vi "Deserialize Data.vi"(8 "error in (no error)":errorcluster, 11 "Flat Data in":string) -> (0 "error out":errorcluster, 3 "Process Data out":T1 {"CAN Frame Array"."payload" format="%x"; "CAN Frame Array"."timestamp" format="%<%.7X\n%x>T"; "CAN Frame Array"."type" items=["CAN Data"=0, "CAN Remote"=1, "CAN Bus Error"=2, "CAN 2.0 Data"=8, "CAN FD Data"=16, "CAN FD+BRS Data"=24, "J1939 Data"=192, "Delay"=224, "Log Trigger"=225, "Start Trigger"=226]; "CAN Frame Array"."identifier" format="%x"})   [LabVIEW 2020, in "NI_ADAS_CAN.lvlib"]
doc: "Version 0.1"
uses:
  NI_ADAS_CAN.lvlib
  Process Data.ctl
  <vilib>/xnet/xnet.llb/XNET Frame CAN.ctl
  <vilib>/xnet/xnet.llb/XNET Frame Type CAN.ctl
  <vilib>/ADAS Record/IODataPEF/CfgMgr/FlatFormat.ctl
  5e2451cd-7b8c-4079-9add-41a600a01e16.vi
  <vilib>/ADAS Record/IODataPEF/Error/Error_SetError.vi
  <vilib>/ADAS Record/IODataPEF/Error/Error_CheckAndSetDllError.vi
  <vilib>/ADAS Record/IODataPEF/Error/ErrorMgr.vi
  <vilib>/ADAS Record/CustomData/_Custom_RegisterType.vi
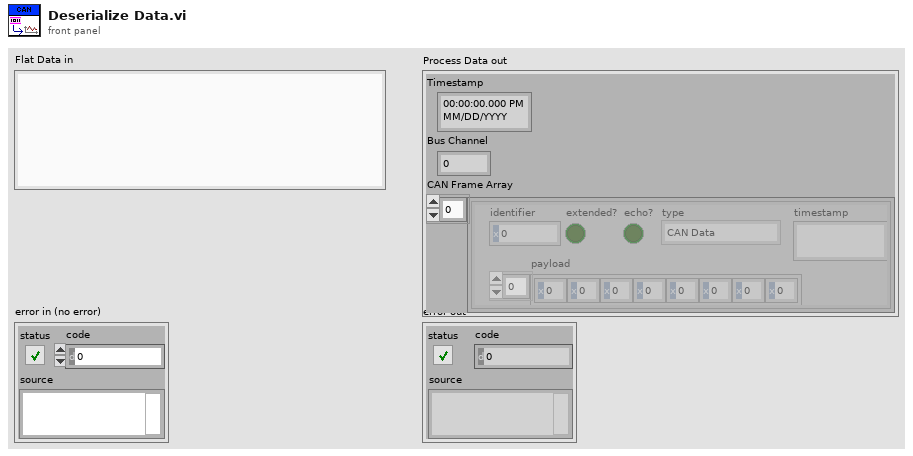
[diagram p1: front panel]
types:
  T1 = typedef "NI_ADAS_CAN.lvlib/Process Data.ctl" = cluster{"Timestamp":timestamp, "Bus Channel":u16, "CAN Frame Array":T2[]}
  T2 = typedef "XNET Frame CAN.ctl" = cluster{"timestamp":timestamp, "payload":u8[], "identifier":u32, "type":T3, "extended?":bool, "echo?":bool}
  T3 = typedef "XNET Frame Type CAN.ctl" = u8
  T4 = typedef "FlatFormat.ctl" = enum32{"Auto", "PEF", "GFB (Apache)", "GFB", "JSON", "Readable JSON", "LV String", "Reserved", "LV Native"}
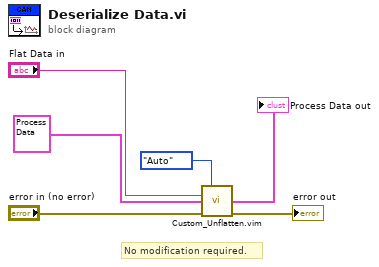
[diagram p0: block diagram]
diagram:
  # "No modification required."
  n1 = call "Custom_Unflatten.vim"("Flat Format"=FlatFormat."Auto", "Flat Data"="Flat Data in", "Data (type/default value)"=T1 {"Timestamp"=timestamp(0 s since 1904-01-01), "Bus Channel"=0, "CAN Frame Array"=[]} ("Byte Array in"), "error in (no error)"="error in (no error)") -> ("Data"=→"Process Data out":T1, "Error (out)"=→"error out":errorcluster)  [unwired: 10 in]
